vi "Digitize I and Q signals v2.vi"(1 "Sample Frequency":u8(ring)=6 items=["4000.0", "5512.50", "6000.00", "6400.00", "8000.00", "11025.00", "12000.00", "12800.00", "16000.00", "22050.00", "24000.00", "25600.00", "32000.00", "44100.00", "48000.00", "51200.00"], 2 "total sampling time":sgl=3.0 min=0 format="%.2f", 5 "file path (dialog if empty)":path=path "d:/mouse") -> ()   [LabVIEW 2022 SP3]
doc: "Scanning siganls from the doppler. WITH NO DISPLAY OF DATA FROM FFT ROUTINE"
uses:
  <vilib>/Waveform/WDTOps.llb/WDT Index Channel DBL.vi
panel:
  in  "Case Constant\n(See Context Help)":bool
  out "frequency":sgl format="%.2f"
  in  "?":cluster{sgl, sgl, sgl, sgl}={44.0, 0.3, 0.0, 0.0} {"?" min=0 max=0.009 step=0.001 scale=0.0..0.009 scale format="%.3f"; "?" min=0 max=0.09 step=0.01 scale=0.0..0.09 scale format="%.2f"; "?" min=0 max=0.9 step=0.1 scale=0.0..0.9 scale format="%.1f"; "?" min=0 max=320 step=1 scale=0.0..320.0}
  out "scan rate":sgl=6000.0 format="%.2f"
  out "number of scans\nto acquire":u32=1024
  out "Intensity Graph":sgl[][](graph)
  in  "change window parameters ?":bool
  in  "stop":bool
  out "Current data file":path
  in  "?":dbl[](array[numeric])=[4000.0, 5512.5, 6000.0, 6400.0, 8000.0, 11025.0, 12000.0, 12800.0, 16000.0, 22050.0, 24000.0, 25600.0, 32000.0, 44100.0, 48000.0, 51200.0] format="%.2f"
  in  "digitize":bool=TRUE
  # "Input Variables"
  # "Change Values"
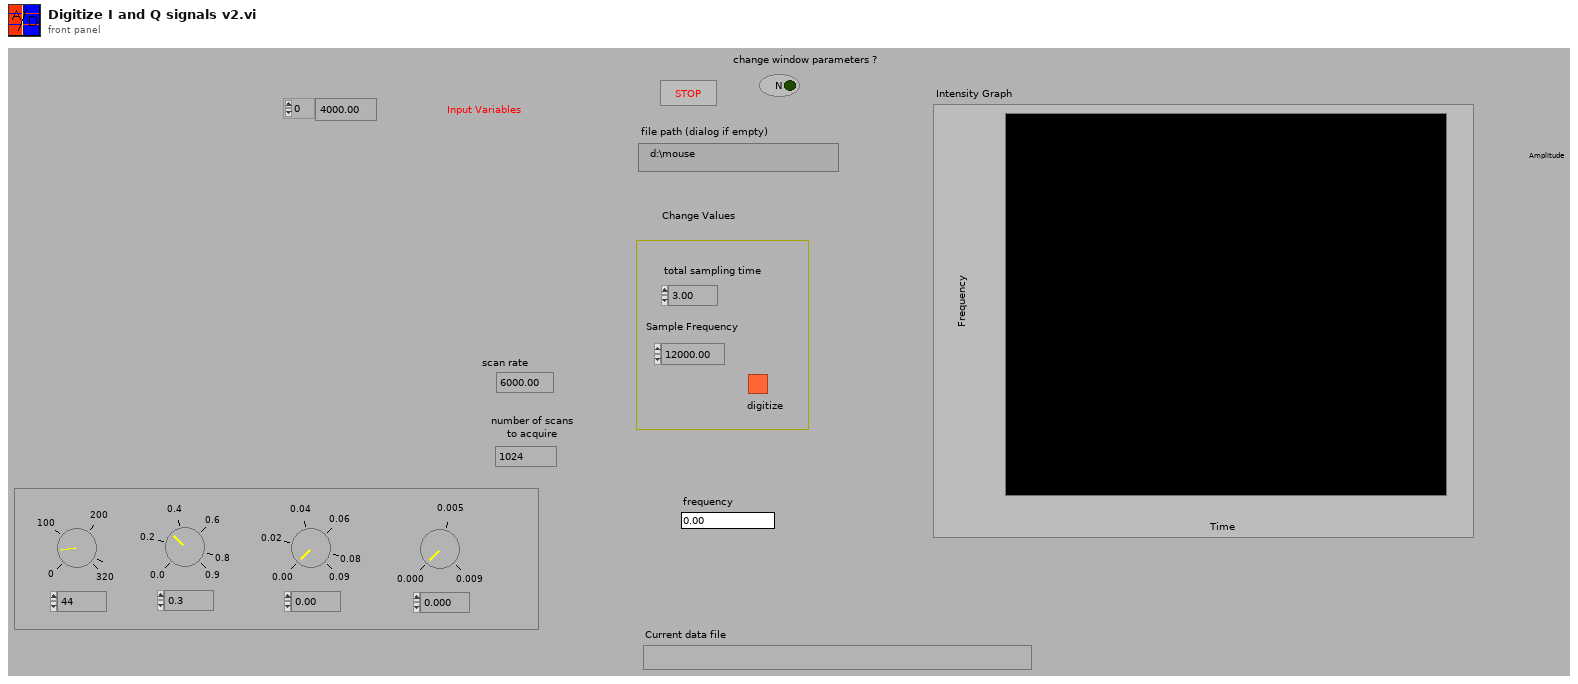
[diagram p1: front panel]
types:
  T1 = cluster{"total time slices":i32, "f0":dbl, "Df":dbl, "Dt":dbl}
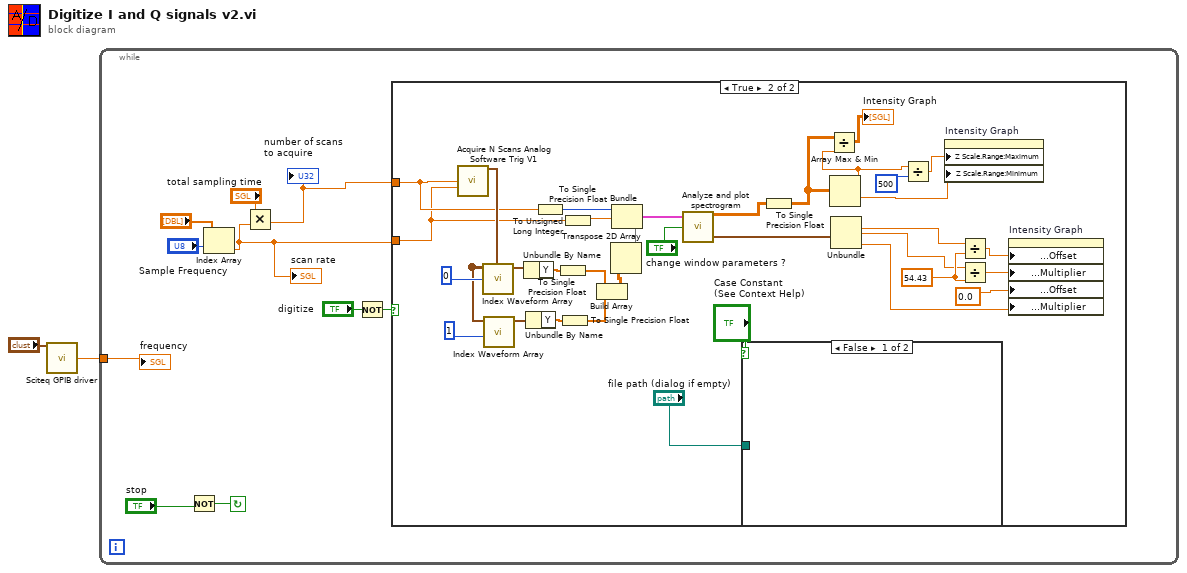
[diagram p0: block diagram]
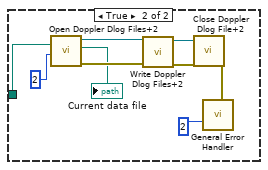
[diagram p3: hidden frame]
diagram:
  n1 = call "Sciteq GPIB driver.vi"(1:"?") -> ("frequency"=w1:sgl)
  n2 = while {
    tunnel: w1 -> [w3]
    stop <- w12 continue-if-true
    n3 = Not(x="stop") -> (.not. x?=w12:bool)
    n4 = Index Array(array="?", index="Sample Frequency") -> (element=w7:dbl)
    "scan rate" <- w7
    n5 = Multiply(x="total sampling time", y=w7) -> (x*y=w6:dbl)
    "number of scans\nto acquire" <- w6
    n6 = Not(x="digitize") -> (.not. x?=w4:bool)
    n7 = case shown="True" w4 {
      tunnel: w6 -> [_ w25]
      tunnel: w7 -> [_ w23]
      frame False {
      }
      frame True {
        w38 = 54.43 ("frequency constant")
        n8 = call "Acquire N Scans Analog Software Trig V1.vi"("number of scans\nto acquire"=w25, "scan rate"=w23) -> ("data"=w28:waveform(dbl)[])  [unwired: 12 in, 1 out]
        n9 = call-poly <vilib>:"Index Waveform Array.vi"("index"=0, "waveform array"=w28) -> ("waveform"=w30:waveform(dbl))  [unwired: 8 in, 1 out]
        n10 = call-poly <vilib>:"Index Waveform Array.vi"("index"=1, "waveform array"=w28) -> ("waveform"=w26:waveform(dbl))  [unwired: 8 in, 1 out]
        n11 = Unbundle By Name(w30) -> ("Y"=w21:dbl[])
        n12 = Unbundle By Name(w26) -> ("Y"=w20:dbl[])
        n13 = To Unsigned Long Integer(number=w25) -> (unsigned 32bit integer=w24:u32)
        n14 = To Single Precision Float(number=w21) -> (single precision float=w18:sgl[])
        n15 = To Single Precision Float(number=w20) -> (single precision float=w17:sgl[])
        n16 = To Single Precision Float(number=w23) -> (single precision float=w22:sgl)
        n17 = Build Array(w18, w17) -> (w16:sgl[][])
        n18 = Transpose 2D Array(2D array=w16) -> (transposed array=w13:sgl[][])
        n19 = Bundle(w24, w22, w13) -> (w19:cluster{u32, sgl, sgl[][]})  [unwired: 1 in]
        n20 = call "Analyze and plot spectrogram .vi"("change window parameters ?"="change window parameters ?", "datalog record"=w19) -> ("Spectrogram Plotting Parameters"=w35:T1, "Spectrogram"=w14:dbl[][])  [unwired: 1 in]
        n21 = case shown="False" "Case Constant\n(See Context Help)" {
          tunnel: "file path (dialog if empty)" -> [_ w50]
          frame False {
          }
          frame True {
            n22 = call "Open Doppler Dlog Files+2.vi"("function (open:0)"=2, "start path  (Not A Path)"=w50) -> ("error out"=w51:errorcluster, "new file path"=→"Current data file":path, "refnum"=w48:refnum<k1>)  [unwired: 6 in, 1 out]
            n23 = call "Write Doppler Dlog Files+2.vi"("error in (no error)"=w51, "refnum"=w48) -> ("error out"=w55:errorcluster, "refnum"=w54:refnum<k1>)  [unwired: 7 in, 1 out]
            n24 = call "Close Doppler Dlog File+2.vi"("error in (no error)"=w55, "refnum"=w54) -> ("error out"=w52:errorcluster)  [unwired: 3 in, 2 out]
            n25 = call <vilib>:"General Error Handler.vi"("type of dialog (OK msg:1)"=2 ("continue or stop message on an error"), "error in (no error)"=w52) -> ()  [unwired: 9 in, 5 out]
          }
        }
        n26 = To Single Precision Float(number=w14) -> (single precision float=w15:sgl[][])
        n27 = Array Max & Min(array=w15) -> (max value=w43:sgl, min value=w39:sgl)  [unwired: 2 out]
        n28 = Divide(x=w15, y=w43) -> (x/y=→"Intensity Graph":sgl[][])
        n29 = Unbundle(w35) -> ("f0"=w37:dbl, "Df"=w36:dbl, "Dt"=w31:dbl)  [unwired: 1 out]
        n30 = Divide(x=w43, y=500) -> (x/y=w40:sgl)
        n31 = property on="Intensity Graph" class="IntGraph (strict)"("Z Scale.Range:Maximum"=w40, "Z Scale.Range:Minimum"=w39) -> ()  [unwired: 2 in, 2 out]
        n32 = Divide(x=w37, y=w38) -> (x/y=w32:dbl)
        n33 = Divide(x=w36, y=w38) -> (x/y=w33:dbl)
        n34 = property on="Intensity Graph" class="IntGraph (strict)"("Y Scale.Offset and Multiplier:Offset"=w32, "Y Scale.Offset and Multiplier:Multiplier"=w33, "X Scale.Offset and Multiplier:Offset"=0.0, "X Scale.Offset and Multiplier:Multiplier"=w31) -> ()  [unwired: 2 in, 2 out]
      }
    }
    "frequency" <- w3
  }
